vi "RT Main - Single Thread.vi"() -> ()   [LabVIEW 2024]
uses:
  Driver/Source/Typedefs/GE 5565PIORC.Typedef.DMA Transfer Spec.ctl
  Driver/Source/Typedefs/GE 5565PIORC.Typedef.DMA Block Descriptor.ctl
  Driver/Source/Typedefs/GE 5565PIORC.Typedef.DMA Block Descriptor Params.ctl
  Driver/Source/Typedefs/GE 5565PIORC.Typedef.DMA Wait Mode.ctl
  <vilib>/Utility/RT CPU Load.ctl
  <vilib>/Platform/TimedLoop/XDataNode/timing_clust.ctl
  <vilib>/Platform/TimedLoop/XDataNode/nitl_modes.ctl
  <vilib>/Platform/TimedLoop/XDataNode/wakeup.ctl
  Driver/Source/GE 5565PIORC.lvclass/GE 5565PIORC.ctl
  Driver/Source/Methods/GE 5565PIORC.DMA.Create Transfer (Block).vi
  Driver/Source/Methods/GE 5565PIORC.DMA.Get Transfer Components (Block).vi
  Driver/Source/Methods/GE 5565PIORC.DMA.Block.Read (DBL).vi
  Driver/Source/Methods/GE 5565PIORC.DMA.Block.Write (DBL).vi
  Driver/Source/Properties/Registers/GE 5565PIORC.Registers.LAS1RR.PCI Address Range.Get.vi
  Driver/Source/Methods/GE 5565PIORC.PXI Interrupts.Enable.vi
  Driver/Source/Properties/Registers/GE 5565PIORC.Registers.DMACSR0.Channel 0 Enable.Set.vi
  Driver/Source/Properties/Registers/GE 5565PIORC.Registers.INTCSR.Local DMA Channel 0 Interrupt Enable.Set.vi
  Driver/Source/Methods/GE 5565PIORC.DMA.Create Transfer (Scatter-Gather).vi
  <vilib>/Utility/error.llb/Clear Errors.vi
  Driver/Source/Properties/Registers/GE 5565PIORC.Registers.DMADPR0.Direction of Transfer.Set.vi
  Driver/Source/Properties/Registers/GE 5565PIORC.Registers.DMASIZ0.DMA Transfer Size.Set.vi
  Driver/Source/Methods/GE 5565PIORC.DMA.Size.vi
  Driver/Source/Properties/Registers/GE 5565PIORC.Registers.DMALADR0.Local Address Register.Set.vi
  Driver/Source/Properties/Registers/GE 5565PIORC.Registers.DMAMODE0.Scatter-Gather Mode.Set.vi
  Driver/Source/Properties/Registers/GE 5565PIORC.Registers.DMAPADR0.PCI Address Register.Set.vi
  Driver/Source/Methods/GE 5565PIORC.DMA.Scatter-Gather.Link Block Descriptors.vi
  Driver/Source/Methods/GE 5565PIORC.DMA.Scatter-Gather.Commit Linked Block Descriptors.vi
  Driver/Source/Properties/Registers/GE 5565PIORC.Registers.DMADPR0.Channel 0 First Descriptor Address.Set.vi
  Driver/Source/Methods/GE 5565PIORC.DMA.Get Transfer Components (Scatter-Gather).vi
  Driver/Source/Properties/Registers/GE 5565PIORC.Registers.DMACSR0.Channel 0 Start.Set.vi
  Driver/Source/Properties/Registers/GE 5565PIORC.Registers.DMACSR0.Channel 0 Clear Interrupt.Set.vi
  Driver/Source/Methods/GE 5565PIORC.DMA.Poll for Done Signal.vi
  Driver/Source/Methods/GE 5565PIORC.PXI Interrupts.Wait for Event.vi
  Driver/Source/Properties/GE 5565PIORC.Read VISA MEMACC.vi
  Driver/Source/Properties/Registers/GE 5565PIORC.Registers.Local Configuration.Read.vi
  Driver/Source/Properties/Registers/GE 5565PIORC.Registers.Local Configuration.Read (U32).vi
  Driver/Source/Properties/Registers/GE 5565PIORC.Registers.Local Configuration.Read (U8).vi
  Driver/Source/Properties/Registers/GE 5565PIORC.Registers.Local Configuration.Write.vi
  Driver/Source/Properties/Registers/GE 5565PIORC.Registers.Local Configuration.Write (U8).vi
  Driver/Source/Methods/GE 5565PIORC.Bit Manipulation.Set Bit.vi
  Driver/Source/Methods/GE 5565PIORC.Bit Manipulation.Set Bit (U8).vi
  Driver/Source/Properties/Registers/GE 5565PIORC.Registers.Local Configuration.Write (U32).vi
  Driver/Source/Methods/GE 5565PIORC.Bit Manipulation.Set Bit (U32).vi
  Driver/Source/Methods/GE 5565PIORC.DMA.Scatter-Gather.Set Descriptor Params.vi
  Driver/Source/Methods/GE 5565PIORC.DMA.Is Done.vi
  Driver/Source/Methods/GE 5565PIORC.Registers.Read.vi
  Driver/Source/Methods/GE 5565PIORC.Registers.Read (U32).vi
  Driver/Source/Methods/GE 5565PIORC.Registers.Read (U8).vi
  Driver/Source/Methods/GE 5565PIORC.Registers.Write.vi
  Driver/Source/Methods/GE 5565PIORC.Registers.Write (U8).vi
  Driver/Source/Methods/GE 5565PIORC.Registers.Write (U32).vi
  Driver/Source/Properties/Registers/GE 5565PIORC.Registers.DMACSR0.Channel 0 Inactive.Get.vi
  Driver/Source/Methods/GE 5565PIORC.Bit Manipulation.Get Bit.vi
  Driver/Source/Methods/GE 5565PIORC.Bit Manipulation.Get Bit (U8).vi
  Driver/Source/Methods/GE 5565PIORC.Round Up to Nearest 8.vi
  Driver/Source/Methods/GE 5565PIORC.Round Up to Nearest 16.vi
  Driver/Source/GE 5565PIORC.lvclass
  <vilib>/platform/TimedLoop/XDataNode/XDataNode.xnode
  <vilib>/Platform/TimedLoop/XDataNode/XDNodeRunTimeDep.lvlib
  <vilib>/NI_Real-Time Target Support.lvlib
panel:
  out "Read Data 2":dbl[](array[numeric])
  out "Prev Read Data":dbl[](array[numeric])
  in  "Read Count (DBLs)":u32
  in  "Write Count (DBLs)":u32
  in  "Reverse Data":bool
  in  "Stop if Different?":bool=TRUE
  out "data out size":i32
  out "Read Size":i32
  out "CPU loads":T1[](array[typedef]) {"ISR (%)" format="%#.2f"; "Idle (%)" format="%#.2f"; "Background (%)" format="%#.2f"; "Normal (%)" format="%#.2f"; "Above Normal (%)" format="%#.2f"; "High (%)" format="%#.2g"; "Timed Structures (%)" format="%#.2g"; "Time Critical (%)" format="%#.2g"; "Total (%)" format="%#.2g"}
  out "Error Code":i32(graph)
  out "Diff Count":i32
  out "Delta T (ms)":u32
  out "Write Timeout":i16(graph)
  out "Read Timeout":i16(graph)
  in  "Write Offset (DBLs)":u32
  in  "Read Offset (DBLs)":u32
  out "Read Data":dbl[][](graph)
  in  "VISA resource name":refnum<visa-resource-name>="PXI17::11::INSTR"
  out "Iteration":i32
  in  "stop":bool
  out "Read Data":dbl[](array[numeric])
  in  "Write Data":dbl[](array[numeric])
  out "Write - DMA Transfer Spec":T2 {"Block Descriptors"."descriptor params"."data ptr (lower)" format="%.0x"; "Block Descriptors"."descriptor params"."data ptr (upper)" format="%.0x"; "Block Descriptors"."descriptor params"."data size" format="%.0x"; "Block Descriptors"."descriptor params"."next descriptor ptr" format="%.0x"; "Block Descriptors"."descriptor size" format="%08x"; "Block Descriptors"."descriptor ptr (RFM)" format="%08x"; "Block Descriptors"."descriptor ptr (VISA)" format="%08x"; "RFM offset" format="%08x"}
  out "Write Time Out?":bool
  out "error out":errorcluster
  out "Read Time Out?":bool
  in  "wait mode (polling)":T5
  out "Read - DMA Transfer Spec":T2 {"Block Descriptors"."descriptor params"."data ptr (lower)" format="%.0x"; "Block Descriptors"."descriptor params"."data ptr (upper)" format="%.0x"; "Block Descriptors"."descriptor params"."data size" format="%.0x"; "Block Descriptors"."descriptor params"."next descriptor ptr" format="%.0x"; "Block Descriptors"."descriptor size" format="%08x"; "Block Descriptors"."descriptor ptr (RFM)" format="%08x"; "Block Descriptors"."descriptor ptr (VISA)" format="%08x"; "RFM offset" format="%08x"}
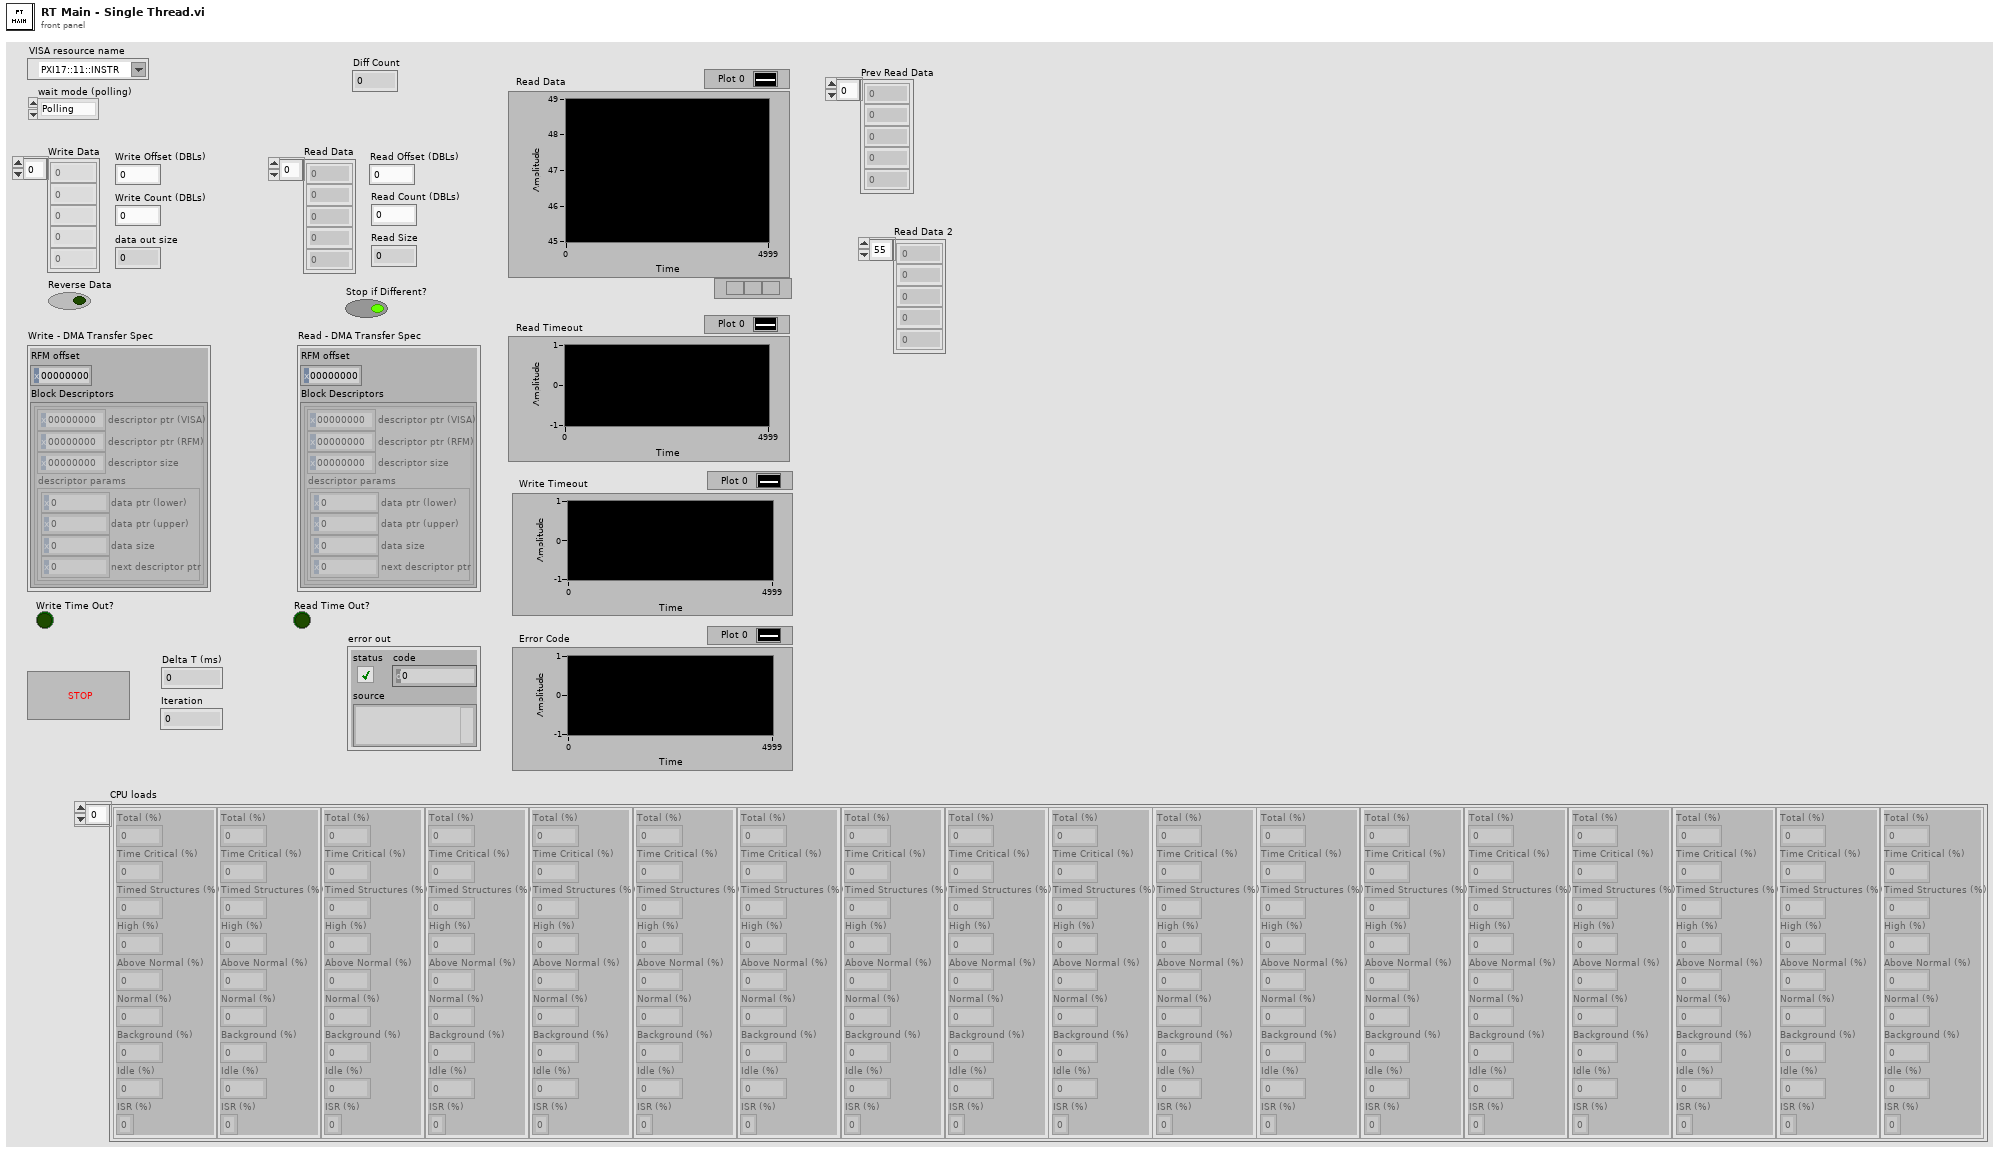
[diagram p1: front panel]
types:
  T1 = typedef "NI_Real-Time Target Support.lvlib/RT CPU Load.ctl" = cluster{"Total (%)":dbl, "Time Critical (%)":dbl, "Timed Structures (%)":dbl, "High (%)":dbl, "Above Normal (%)":dbl, "Normal (%)":dbl, "Background (%)":dbl, "Idle (%)":dbl, "ISR (%)":dbl}
  T2 = typedef "GE 5565PIORC.lvclass/GE 5565PIORC.Typedef.DMA Transfer Spec.ctl" = cluster{"RFM offset":u32, "Block Descriptors":T3[]}
  T3 = typedef "GE 5565PIORC.lvclass/GE 5565PIORC.Typedef.DMA Block Descriptor.ctl" = cluster{"descriptor ptr (VISA)":u32, "descriptor ptr (RFM)":u32, "descriptor size":u32, "descriptor params":T4}
  T4 = typedef "GE 5565PIORC.lvclass/GE 5565PIORC.Typedef.DMA Block Descriptor Params.ctl" = cluster{"data ptr (lower)":u32, "data ptr (upper)":u32, "data size":u32, "next descriptor ptr":u32}
  T5 = typedef "GE 5565PIORC.lvclass/GE 5565PIORC.Typedef.DMA Wait Mode.ctl" = enum16{"Polling", "Interrupt"}
  T6 = typedef "XDNodeRunTimeDep.lvlib/timing_clust.ctl" = cluster{"Expected End [f-1]":u64, "Actual End [f-1]":u64, "Finished Late? [f-1]":bool, "Expected End [i-1]":u64, "Actual End [i-1]":u64, "Finished Late? [i-1]":bool, "Expected Start [i]":u64, "Actual Start [i]":u64, "Expected Start [f]":u64, "Actual Start [f]":u64, "Source Name":string, "Structure Name":string, "Period":i64, "Deadline":i64, "Offset":i64, "Start":i64, "Priority":i32, "Timeout":i32, "Mode":T7, "Wakeup Reason":T8, "Error":errorcluster, "Source Type":string, "Secondary Source Type":string, "Global End Time":u64, "Global Start Time":u64, "Frame Duration":u64, "Iteration Duration":u64, "Assigned CPU":i32, "I/O Scan Engine Mode":u32}
  T7 = typedef "XDNodeRunTimeDep.lvlib/nitl_modes.ctl" = enum32{"No Change", "Process missed periods, maintain original phase", "Discard missed periods, maintain original phase", "Process missed periods, ignore original phase", "Discard missed periods, ignore original phase"}
  T8 = typedef "XDNodeRunTimeDep.lvlib/wakeup.ctl" = enum32{"Normal", "Aborted", "Asynchronous wakeup", "Timing source error", "Timed loop error", "Timeout"}
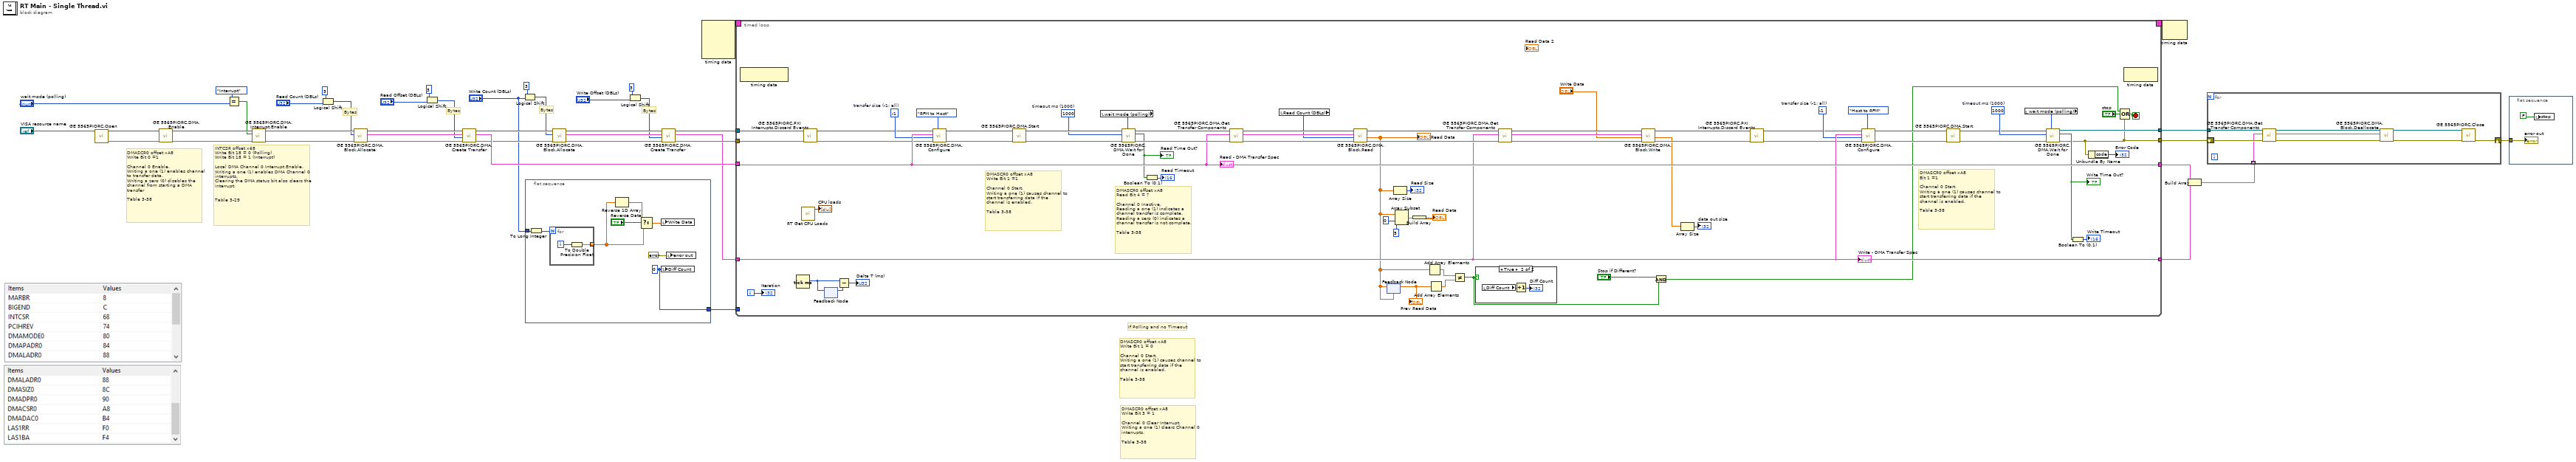
[diagram p0: block diagram]
diagram:
  # "Bytes"
  # "Bytes"
  # "Bytes"
  # "Bytes"
  # "If Polling and no Timeout"
  # "DMASCR0 offset xA8\nWrite Bit 3 = 1\n\nChannel 0 Clear Interrupt. \nWriting a one (1) clears Channel 0 interrupts.\n\nTable 3-38"
  # "DMASCR0 offset xA8\nWrite Bit 1 = 0\n\nChannel 0 Start. \nWriting a one (1) causes channel to start transferring data if the \nchannel is enabled.\n\nTable 3-38"
  # "INTCSR offset x68\nWrite Bit 18 = 0 (Polling)\nWrite Bit 18 = 1 (Interrupt)\n\nLocal DMA Channel 0 Interrupt Enable. \nWriting a one (1) enables DMA Channel 0 interrupts. \nClearing the DMA status bit also clears the interrupt.\n\n\nTable 3-29"
  # "DMASCR0 offset xA8\nWrite Bit 0 =1\n\nChannel 0 Enable. \nWriting a one (1) enables channel to transfer data. \nWriting a zero (0) disables the channel from starting a DMA \ntransfer\n\nTable 3-38"
  n1 = call "GE 5565PIORC.Open.vi"("VISA resource name"="VISA resource name") -> ("error out"=w42:errorcluster, "GE 5565PIORC"=w43:refnum<class "GE 5565PIORC.lvclass">)  [unwired: 9 in]
  n2 = call "GE 5565PIORC.DMA.Enable.vi"("error in (no error)"=w42, "GE 5565PIORC in"=w43) -> ("error out"=w38:errorcluster, "GE 5565PIORC out"=w39:refnum<class "GE 5565PIORC.lvclass">)  [unwired: 8 in]
  n3 = Equal?(x=GE_5565PIORC.Typedef.DMA_Wait_Mode."Interrupt" ("wait mode (polling)"), y="wait mode (polling)") -> (x = y?=w28:bool)
  n4 = call "GE 5565PIORC.DMA.Interrupt.Enable.vi"("error in (no error)"=w38, "enable (T)"=w28, "GE 5565PIORC in"=w39) -> ("error out"=w31:errorcluster, "GE 5565PIORC out"=w32:refnum<class "GE 5565PIORC.lvclass">)  [unwired: 7 in]
  n5 = Logical Shift(y=i16 3, x="Read Count (DBLs)") -> (x << y=w10:u32)
  n6 = call "GE 5565PIORC.DMA.Block.Allocate.vi"("error in (no error)"=w31, "size in bytes"=w10, "GE 5565PIORC in"=w32) -> ("error out"=w41:errorcluster, "Block Descriptor"=w40:T3, "GE 5565PIORC out"=w33:refnum<class "GE 5565PIORC.lvclass">)  [unwired: 6 in]
  n7 = Logical Shift(y=i16 3, x="Read Offset (DBLs)") -> (x << y=w4:u32)
  n8 = call-poly "GE 5565PIORC.DMA.Create Transfer.vi"("error in (no error)"=w41, "RFM offset"=w4, "Block Descriptor"=w40, "GE 5565PIORC in"=w33) -> ("error out"=w23:errorcluster, "DMA Transfer Spec"=w35:T2, "GE 5565PIORC out"=w24:refnum<class "GE 5565PIORC.lvclass">)  [unwired: 4 in, 1 out]
  n9 = Logical Shift(y=i16 3, x="Write Count (DBLs)") -> (x << y=w7:u32)
  n10 = flat-sequence {
    tunnel: [w51] -> w13
    tunnel: "Write Count (DBLs)" -> [w45]
    frame #0 {
      w51 = 0 ("Diff Count")
      n11 = To Long Integer(number=w45) -> (32bit integer=w46:i32)
      n12 = for {
        N: w46 -> [_]
        tunnel: [w52] -> w49 mode=indexing
        i -> [w53]
        n13 = To Double Precision Float(number=w53) -> (double precision float=w52:dbl)
      }
      n14 = Reverse 1D Array(array=w49) -> (reversed array=w50:dbl[])
      n15 = Select(t=w50, s="Reverse Data", f=w49) -> (s? t:f=w47:dbl[])
      n16 = local write "Write Data"(w47) -> ()
      n17 = local write "Diff Count"(w51) -> ()
      n18 = local write "error out"(errorcluster {"status"=FALSE, "code"=0, "source"=""} ("error out")) -> ()
    }
  }
  n19 = call "GE 5565PIORC.DMA.Block.Allocate.vi"("error in (no error)"=w23, "size in bytes"=w7, "GE 5565PIORC in"=w24) -> ("error out"=w26:errorcluster, "Block Descriptor"=w25:T3, "GE 5565PIORC out"=w27:refnum<class "GE 5565PIORC.lvclass">)  [unwired: 6 in]
  n20 = Logical Shift(y=i16 3, x="Write Offset (DBLs)") -> (x << y=w1:u32)
  n21 = call-poly "GE 5565PIORC.DMA.Create Transfer.vi"("error in (no error)"=w26, "RFM offset"=w1, "Block Descriptor"=w25, "GE 5565PIORC in"=w27) -> ("error out"=w21:errorcluster, "DMA Transfer Spec"=w19:T2, "GE 5565PIORC out"=w22:refnum<class "GE 5565PIORC.lvclass">)  [unwired: 4 in, 1 out]
  n22 = node-c288() -> (w37:T6)  [unwired: 4 in]
  n23 = timed-loop {
    timing: w37 -> [_]
    timing-out: [_] -> w36
    tunnel: w22 -> [w102]
    tunnel: w21 -> [w101]
    tunnel: w35 -> [w112]
    tunnel: [w112] -> w16
    tunnel: w19 -> [w84]
    tunnel: [w76] -> w18
    tunnel: [w85] -> w17
    tunnel: [w84] -> w15
    tunnel: w13 -> [_]
    i -> [w109]
    stop <- w110 stop-if-true
    w69 = -1  # transfer size (-1: all)
    w74 = -1  # transfer size (-1: all)
    w96 = u32 1000  # timeout ms (1000)
    w111 = u32 1000  # timeout ms (1000)
    # "DMASCR0 offset xA8\nRead Bit 4 = ?\n\nChannel 0 Inactive. \nReading a one (1) indicates a channel transfer is complete. \nReading a zero (0) indicates a channel transfer is not complete.\n\nTable 3-38"
    # "DMASCR0 offset xA8\nBit 1 =1\n\nChannel 0 Start. \nWriting a one (1) causes channel to start transferring data if the \nchannel is enabled.\n\nTable 3-38"
    # "DMASCR0 offset xA8\nWrite Bit 1 =1\n\nChannel 0 Start. \nWriting a one (1) causes channel to start transferring data if the \nchannel is enabled.\n\nTable 3-38"
    n24 = node-c288() -> ()  [unwired: 1 in, 1 out]
    n25 = Tick Count (ms)() -> (millisecond timer value=w83:u32)
    n26 = call <vilib>:"RT Get CPU Loads.vi"() -> ("CPU loads"=→"CPU loads":T1[])  [unwired: 10 in, 1 out]
    n27 = call "GE 5565PIORC.PXI Interrupts.Discard Events.vi"("error in (no error)"=w101, "GE 5565PIORC in"=w102) -> ("error out"=w67:errorcluster, "GE 5565PIORC out"=w68:refnum<class "GE 5565PIORC.lvclass">)  [unwired: 8 in]
    n28 = feedback-in #1(w83) -> ()
    n29 = feedback #1() -> (w82:u32)  [unwired: 1 in]
    n30 = Subtract(x=w83, y=w82) -> (x-y=→"Delta T (ms)":u32)
    n31 = call "GE 5565PIORC.DMA.Configure.vi"("transfer direction"=enum16{"Host to RFM", "RFM to Host"}."RFM to Host", "error in (no error)"=w67, "transfer size (-1: all)"=w69, "DMA Transfer Spec"=w112, "GE 5565PIORC in"=w68) -> ("error out"=w117:errorcluster, "GE 5565PIORC out"=w119:refnum<class "GE 5565PIORC.lvclass">)  [unwired: 5 in]
    n32 = call "GE 5565PIORC.DMA.Start.vi"("error in (no error)"=w117, "GE 5565PIORC in"=w119) -> ("error out"=w116:errorcluster, "GE 5565PIORC out"=w118:refnum<class "GE 5565PIORC.lvclass">)  [unwired: 8 in]
    n33 = local read "wait mode (polling)"() -> (w115:T5)
    n34 = call "GE 5565PIORC.DMA.Wait for Done.vi"("wait mode (polling)"=w115, "error in (no error)"=w116, "timeout ms (1000)"=w111, "GE 5565PIORC in"=w118) -> ("error out"=w113:errorcluster, "timed out?"=w104:bool, "GE 5565PIORC out"=w114:refnum<class "GE 5565PIORC.lvclass">)  [unwired: 5 in]
    "Read Time Out?" <- w104
    n35 = Boolean To (0,1)(Boolean=w104) -> (0, 1=→"Read Timeout":i16)
    n36 = call-poly "GE 5565PIORC.DMA.Get Transfer Components.vi"("error in (no error)"=w113, "DMA Transfer Spec in"=w112, "GE 5565PIORC in"=w114) -> ("error out"=w106:errorcluster, "Block Descriptor"=w105:T3, "GE 5565PIORC out"=w107:refnum<class "GE 5565PIORC.lvclass">)  [unwired: 5 in, 1 out]
    n37 = local read "Read Count (DBLs)"() -> (w54:u32)
    n38 = call-poly "GE 5565PIORC.DMA.Block.Read.vi"("error in (no error)"=w106, "count"=w54, "Block Descriptor in"=w105, "GE 5565PIORC in"=w107) -> ("error out"=w88:errorcluster, "data out"=w57:dbl[], "GE 5565PIORC out"=w87:refnum<class "GE 5565PIORC.lvclass">)  [unwired: 4 in, 1 out]
    "Read Data" <- w57
    n39 = feedback-in #2(w57) -> ()
    n40 = feedback #2(w57) -> (w56:dbl[])
    "Prev Read Data" <- w56
    n41 = Array Size(array=w57) -> (size(s)=→"Read Size":i32)
    n42 = Array Subset(array=w57, index=0, length=5) -> (w77:dbl[])
    n43 = Build Array(w77) -> (→"Read Data":dbl[][])
    n44 = Add Array Elements(numeric array=w57) -> (sum=w59:dbl)
    n45 = Add Array Elements(numeric array=w56) -> (sum=w58:dbl)
    n46 = Not Equal?(x=w59, y=w58) -> (x != y?=w61:bool)
    n47 = case shown="True" w61 {
      frame False {
      }
      frame True {
        n48 = local read "Diff Count"() -> (w121:i32)
        n49 = Increment(x=w121) -> (x+1=→"Diff Count":i32)
      }
    }
    n50 = call-poly "GE 5565PIORC.DMA.Get Transfer Components.vi"("error in (no error)"=w88, "DMA Transfer Spec in"=w84, "GE 5565PIORC in"=w87) -> ("error out"=w90:errorcluster, "Block Descriptor"=w89:T3, "GE 5565PIORC out"=w86:refnum<class "GE 5565PIORC.lvclass">)  [unwired: 5 in, 1 out]
    n51 = call-poly "GE 5565PIORC.DMA.Block.Write.vi"("error in (no error)"=w90, "data"="Write Data", "Block Descriptor in"=w89, "GE 5565PIORC in"=w86) -> ("error out"=w98:errorcluster, "data out"=w55:dbl[], "GE 5565PIORC out"=w97:refnum<class "GE 5565PIORC.lvclass">)  [unwired: 4 in, 1 out]
    n52 = And(x="Stop if Different?", y=w61) -> (x .and. y?=w60:bool)
    n53 = Array Size(array=w55) -> (size(s)=→"data out size":i32)
    n54 = call "GE 5565PIORC.PXI Interrupts.Discard Events.vi"("error in (no error)"=w98, "GE 5565PIORC in"=w97) -> ("error out"=w71:errorcluster, "GE 5565PIORC out"=w72:refnum<class "GE 5565PIORC.lvclass">)  [unwired: 8 in]
    n55 = call "GE 5565PIORC.DMA.Configure.vi"("transfer direction"=enum16{"Host to RFM", "RFM to Host"}."Host to RFM", "error in (no error)"=w71, "transfer size (-1: all)"=w74, "DMA Transfer Spec"=w84, "GE 5565PIORC in"=w72) -> ("error out"=w91:errorcluster, "GE 5565PIORC out"=w93:refnum<class "GE 5565PIORC.lvclass">)  [unwired: 5 in]
    n56 = call "GE 5565PIORC.DMA.Start.vi"("error in (no error)"=w91, "GE 5565PIORC in"=w93) -> ("error out"=w92:errorcluster, "GE 5565PIORC out"=w94:refnum<class "GE 5565PIORC.lvclass">)  [unwired: 8 in]
    n57 = local read "wait mode (polling)"() -> (w95:T5)
    n58 = call "GE 5565PIORC.DMA.Wait for Done.vi"("wait mode (polling)"=w95, "error in (no error)"=w92, "timeout ms (1000)"=w96, "GE 5565PIORC in"=w94) -> ("error out"=w76:errorcluster, "timed out?"=w99:bool, "GE 5565PIORC out"=w85:refnum<class "GE 5565PIORC.lvclass">)  [unwired: 5 in]
    "Write Time Out?" <- w99
    n59 = Boolean To (0,1)(Boolean=w99) -> (0, 1=→"Write Timeout":i16)
    n60 = Unbundle By Name(w76) -> ("code"=→"Error Code":i32)
    n61 = Compound Arithmetic op=OR(w60, "stop", w76) -> (w110:bool)
    n62 = node-c288() -> ()  [unwired: 1 in, 1 out]
    "Read - DMA Transfer Spec" <- w112
    "Iteration" <- w109
    "Write - DMA Transfer Spec" <- w84
  }
  n63 = node-c288(w36) -> ()  [unwired: 1 out]
  n64 = Build Array(w16, w15) -> (w14:T2[])
  n65 = for {
    tunnel: w17 -> [w125]
    shift-right: [w127] -> w20
    shift-left: w18 -> [w126]
    tunnel: w14 -> [w124] mode=indexing
    n66 = call-poly "GE 5565PIORC.DMA.Get Transfer Components.vi"("error in (no error)"=w126, "DMA Transfer Spec in"=w124, "GE 5565PIORC in"=w125) -> ("error out"=w130:errorcluster, "Block Descriptor"=w131:T3, "GE 5565PIORC out"=w132:refnum<class "GE 5565PIORC.lvclass">)  [unwired: 5 in, 1 out]
    n67 = call "GE 5565PIORC.DMA.Block.Deallocate.vi"("error in (no error)"=w130, "Block Descriptor"=w131, "GE 5565PIORC in"=w132) -> ("error out"=w128:errorcluster, "GE 5565PIORC out"=w129:refnum<class "GE 5565PIORC.lvclass">)  [unwired: 7 in]
    n68 = call "GE 5565PIORC.Close.vi"("error in (no error)"=w128, "GE 5565PIORC in"=w129) -> ("error out"=w127:errorcluster)  [unwired: 8 in, 1 out]
  }
  n69 = flat-sequence {
    tunnel: w20 -> [w134]
    frame #0 {
      n70 = local write "stop"(FALSE) -> ()
      "error out" <- w134
    }
  }
